vi "cs_RS232TMC_read.vi"(8 "error in (no error)":errorcluster, 11 "Variant In":variant) -> (0 "error out":errorcluster, 2 "string":string, 3 "variant":variant)   [LabVIEW 2024]
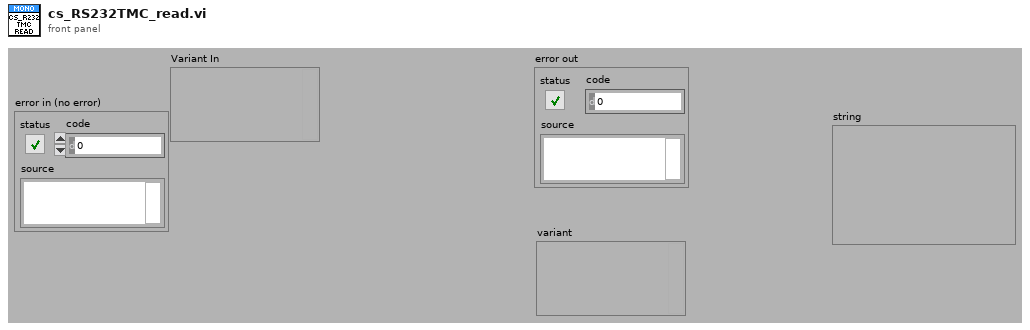
[diagram p1: front panel]
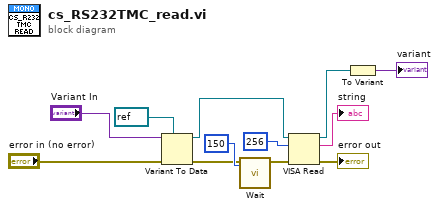
[diagram p0: block diagram]
diagram:
  n1 = Variant To Data(error in="error in (no error)", type=refnum<visa-resource-name> refnum ("VISA resource name"), Variant="Variant In") -> (data=w5:refnum<visa-resource-name>, error out=w7:errorcluster)
  n2 = call "Wait.vi"("milliseconds to wait"=u32 150, "Error In"=w7) -> ("Error Out"=w11:errorcluster)  [unwired: 9 in]
  n3 = VISA Read(VISA resource name=w5, byte count=u32 256, error in (no error)=w11) -> (VISA resource name out=w4:refnum<visa-resource-name>, read buffer=→"string":string, error out=→"error out":errorcluster)  [unwired: 1 out]
  n4 = To Variant(anything=w4) -> (Variant=→"variant":variant)
